vi "MDrive_Get_Parameter.vi"(4 "error in":errorcluster, 6 "Get Parameter":T1, 7 "VISA resource name in":refnum<visa-resource-name>) -> (0 "error out":errorcluster, 1 "Parameter Data Numeric":i32, 2 "Parameter Data String":string, 3 "VISA resource name out":refnum<visa-resource-name>)   [LabVIEW 2013]
uses:
  Get Parameter.ctl
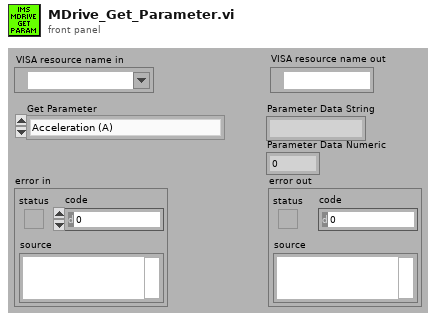
[diagram p1: front panel]
types:
  T1 = typedef "Get Parameter.ctl" = enum16{"Acceleration (A)", "Baud Rate (BD)", "Busy Flag (BY)", "Counter 1 (C1)", "Counter 2 (C2)", "Check Sum Enable (CK)", "Clock Mode (CM)", "Clock Mode Ratio (CR)", "Clock Mode Out Step Width (CW)", "Deceleration (D)", "Digital Filtering, Input 1 (D1)", "Digital Filtering, Input 2 (D2)", "Digital Filtering, Input 3 (D3)", "Digital Filtering, Input 4 (D4)", "Digital Filtering, Input 5 (D5)", "Digital Filtering, Input 9 (D9)", "Digital Filtering, Input 10 (D10)", "Digital Filtering, Input 11 (D11)", "Digital Filtering, Input 12 (D12)", "Deadband (DB)", "Enable/Disable Drive (DE)", "Device Name (DN)", "End Program Execution (E)", "Encoder Function Enable (EE)", "Encoder Lines (EL)", "Error Flag (EF)", "Error Variable (ER)", "Echo Mode (EM)", "Escape (ES)", "Execute Program at Address (EX)", "Hold Current (HC)", "Hold Current Delay Time (HI)", "Input 1 (I1)", "Input 2 (I2)", "Input 3 (I3)", "Input 4 (I4)", "Input 5 Analog (I5)", "Input 6 Encoder Index (I6)", "Input 9 (I9)", "Input 10 (I10)", "Input 11 (I11)", "Input 12 (I12)", "Input Low Byte (1-4) (IL)", "Input High Byte (9-12) (IH)", "Inputs Total (1-4,9-12) (IN)", "Internal Temperature (IT)", "Jog Enable (JE)", "Limit Stop Mode (LM)", "MicroStepping Select (MS)", "Motor Settling Delay Time (MT)", "Moving Flag (MV)", "Output 1 (O1)", "Output 2 (O2)", "Output 3 (O3)", "Output 4 (O4)", "Output 9 (O9)", "Output 10 (O10)", "Output 11 (O11)", "Output 12 (O12)", "Output High Byte (9-12) (OH)", "Output Low Byte (1-4) (OL)", "Output Total (1-4 and 9-12) (OT)", "Position Captured at Trip (PC)", "Position Maintenance (PM)", "Part Number (PN)", "Party Mode (PY)", "Register 1 (R1)", "Register 2 (R2)", "Register 3 (R3)", "Register 4 (R4)", "Run Current (RC)", "Serial Number (SN)", "Stall Flag (ST)", "Stall Factor (SF)", "Stall Mode Set (SM)", "User Variables (UV)", "Velocity (V)", "Velocity Changing Flag (VC)", "Velocity Initial (VI)", "Version, Firmware (VR)", "Velocity Maximum (VM)"}
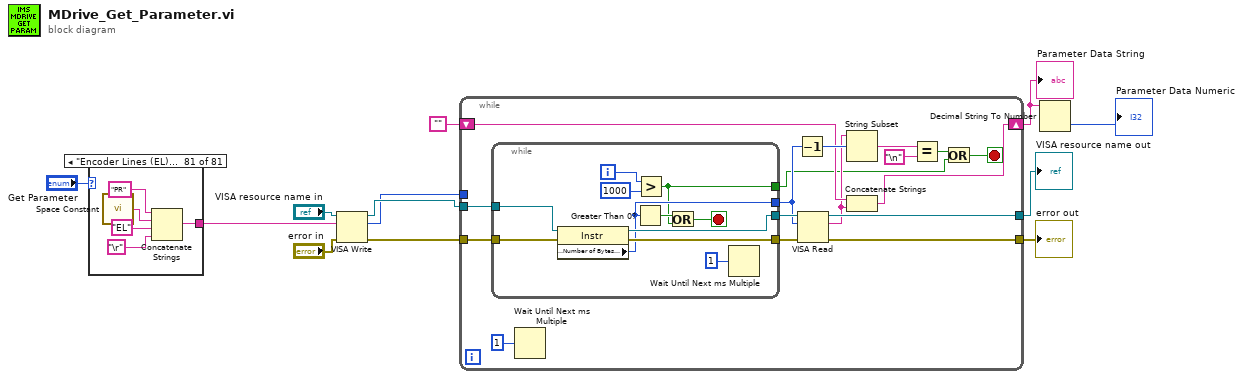
[diagram p0: block diagram]
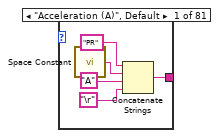
[diagram p2: hidden frame]
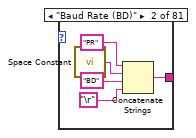
[diagram p3: hidden frame]
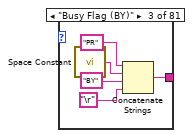
[diagram p4: hidden frame]
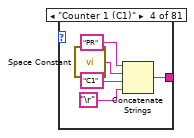
[diagram p5: hidden frame]
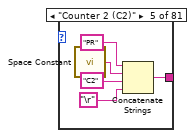
[diagram p6: hidden frame]
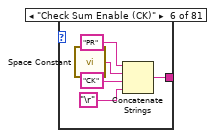
[diagram p7: hidden frame]
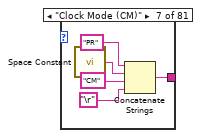
[diagram p8: hidden frame]
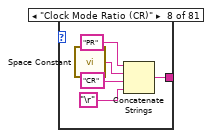
[diagram p9: hidden frame]
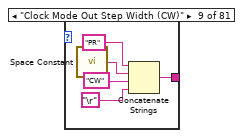
[diagram p10: hidden frame]
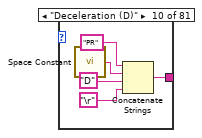
[diagram p11: hidden frame]
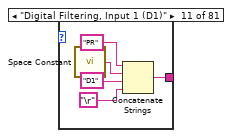
[diagram p12: hidden frame]
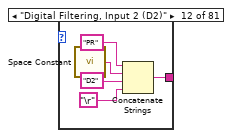
[diagram p13: hidden frame]
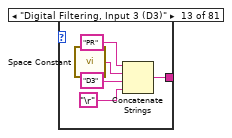
[diagram p14: hidden frame]
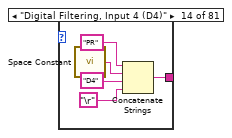
[diagram p15: hidden frame]
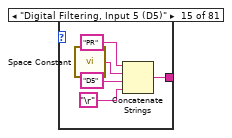
[diagram p16: hidden frame]
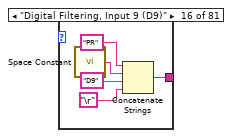
[diagram p17: hidden frame]
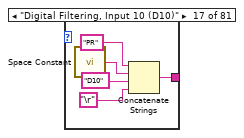
[diagram p18: hidden frame]
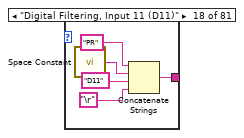
[diagram p19: hidden frame]
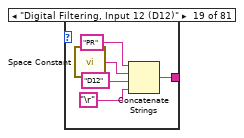
[diagram p20: hidden frame]
diagram:
  n1 = case shown="\"Encoder Lines (EL)\"" "Get Parameter" {
    tunnel: [w13 w18 w23 w28 w33 w38 w43 w48 w53 w58 w63 w68 w73 w78 w83 w88 w93 w98 w103 w108 w113 w118 w123 w128 w133 w138 w143 w148 w153 w158 w163 w168 w173 w178 w183 w188 w193 w198 w203 w208 w213 w218 w223 w228 w233 w238 w243 w248 w253 w258 w263 w268 w273 w278 w283 w288 w293 w298 w303 w308 w313 w318 w323 w328 w333 w338 w343 w348 w353 w358 w363 w368 w373 w378 w383 w388 w393 w398 w403 w408 w413] -> w3
    frame "Acceleration (A)", Default {
      n2 = call <vilib>:"Space Constant.vi"() -> ("String"=w16:string)
      n3 = Concatenate Strings("PR" ("string"), w16, "A" ("string"), "\r") -> (w13:string)
    }
    frame "Baud Rate (BD)" {
      n4 = call <vilib>:"Space Constant.vi"() -> ("String"=w21:string)
      n5 = Concatenate Strings("PR" ("string"), w21, "BD" ("string"), "\r") -> (w18:string)
    }
    frame "Busy Flag (BY)" {
      n6 = call <vilib>:"Space Constant.vi"() -> ("String"=w26:string)
      n7 = Concatenate Strings("PR" ("string"), w26, "BY" ("string"), "\r") -> (w23:string)
    }
    frame "Counter 1 (C1)" {
      n8 = call <vilib>:"Space Constant.vi"() -> ("String"=w31:string)
      n9 = Concatenate Strings("PR" ("string"), w31, "C1" ("string"), "\r") -> (w28:string)
    }
    frame "Counter 2 (C2)" {
      n10 = call <vilib>:"Space Constant.vi"() -> ("String"=w36:string)
      n11 = Concatenate Strings("PR" ("string"), w36, "C2" ("string"), "\r") -> (w33:string)
    }
    frame "Check Sum Enable (CK)" {
      n12 = call <vilib>:"Space Constant.vi"() -> ("String"=w41:string)
      n13 = Concatenate Strings("PR" ("string"), w41, "CK" ("string"), "\r") -> (w38:string)
    }
    frame "Clock Mode (CM)" {
      n14 = call <vilib>:"Space Constant.vi"() -> ("String"=w46:string)
      n15 = Concatenate Strings("PR" ("string"), w46, "CM" ("string"), "\r") -> (w43:string)
    }
    frame "Clock Mode Ratio (CR)" {
      n16 = call <vilib>:"Space Constant.vi"() -> ("String"=w51:string)
      n17 = Concatenate Strings("PR" ("string"), w51, "CR" ("string"), "\r") -> (w48:string)
    }
    frame "Clock Mode Out Step Width (CW)" {
      n18 = call <vilib>:"Space Constant.vi"() -> ("String"=w56:string)
      n19 = Concatenate Strings("PR" ("string"), w56, "CW" ("string"), "\r") -> (w53:string)
    }
    frame "Deceleration (D)" {
      n20 = call <vilib>:"Space Constant.vi"() -> ("String"=w61:string)
      n21 = Concatenate Strings("PR" ("string"), w61, "D" ("string"), "\r") -> (w58:string)
    }
    frame "Digital Filtering, Input 1 (D1)" {
      n22 = call <vilib>:"Space Constant.vi"() -> ("String"=w66:string)
      n23 = Concatenate Strings("PR" ("string"), w66, "D1" ("string"), "\r") -> (w63:string)
    }
    frame "Digital Filtering, Input 2 (D2)" {
      n24 = call <vilib>:"Space Constant.vi"() -> ("String"=w71:string)
      n25 = Concatenate Strings("PR" ("string"), w71, "D2" ("string"), "\r") -> (w68:string)
    }
    frame "Digital Filtering, Input 3 (D3)" {
      n26 = call <vilib>:"Space Constant.vi"() -> ("String"=w76:string)
      n27 = Concatenate Strings("PR" ("string"), w76, "D3" ("string"), "\r") -> (w73:string)
    }
    frame "Digital Filtering, Input 4 (D4)" {
      n28 = call <vilib>:"Space Constant.vi"() -> ("String"=w81:string)
      n29 = Concatenate Strings("PR" ("string"), w81, "D4" ("string"), "\r") -> (w78:string)
    }
    frame "Digital Filtering, Input 5 (D5)" {
      n30 = call <vilib>:"Space Constant.vi"() -> ("String"=w86:string)
      n31 = Concatenate Strings("PR" ("string"), w86, "D5" ("string"), "\r") -> (w83:string)
    }
    frame "Digital Filtering, Input 9 (D9)" {
      n32 = call <vilib>:"Space Constant.vi"() -> ("String"=w91:string)
      n33 = Concatenate Strings("PR" ("string"), w91, "D9" ("string"), "\r") -> (w88:string)
    }
    frame "Digital Filtering, Input 10 (D10)" {
      n34 = call <vilib>:"Space Constant.vi"() -> ("String"=w96:string)
      n35 = Concatenate Strings("PR" ("string"), w96, "D10" ("string"), "\r") -> (w93:string)
    }
    frame "Digital Filtering, Input 11 (D11)" {
      n36 = call <vilib>:"Space Constant.vi"() -> ("String"=w101:string)
      n37 = Concatenate Strings("PR" ("string"), w101, "D11" ("string"), "\r") -> (w98:string)
    }
    frame "Digital Filtering, Input 12 (D12)" {
      n38 = call <vilib>:"Space Constant.vi"() -> ("String"=w106:string)
      n39 = Concatenate Strings("PR" ("string"), w106, "D12" ("string"), "\r") -> (w103:string)
    }
    frame "Deadband (DB)" {
      n40 = call <vilib>:"Space Constant.vi"() -> ("String"=w111:string)
      n41 = Concatenate Strings("PR" ("string"), w111, "DB" ("string"), "\r") -> (w108:string)
    }
    frame "Enable/Disable Drive (DE)" {
      n42 = call <vilib>:"Space Constant.vi"() -> ("String"=w116:string)
      n43 = Concatenate Strings("PR" ("string"), w116, "DE" ("string"), "\r") -> (w113:string)
    }
    frame "Device Name (DN)" {
      n44 = call <vilib>:"Space Constant.vi"() -> ("String"=w121:string)
      n45 = Concatenate Strings("PR" ("string"), w121, "DN" ("string"), "\r") -> (w118:string)
    }
    frame "End Program Execution (E)" {
      n46 = call <vilib>:"Space Constant.vi"() -> ("String"=w126:string)
      n47 = Concatenate Strings("PR" ("string"), w126, "E" ("string"), "\r") -> (w123:string)
    }
    frame "Encoder Function Enable (EE)" {
      n48 = call <vilib>:"Space Constant.vi"() -> ("String"=w131:string)
      n49 = Concatenate Strings("PR" ("string"), w131, "EE" ("string"), "\r") -> (w128:string)
    }
    frame "Error Flag (EF)" {
      n50 = call <vilib>:"Space Constant.vi"() -> ("String"=w136:string)
      n51 = Concatenate Strings("PR" ("string"), w136, "EF" ("string"), "\r") -> (w133:string)
    }
    frame "Error Variable (ER)" {
      n52 = call <vilib>:"Space Constant.vi"() -> ("String"=w141:string)
      n53 = Concatenate Strings("PR" ("string"), w141, "ER" ("string"), "\r") -> (w138:string)
    }
    frame "Echo Mode (EM)" {
      n54 = call <vilib>:"Space Constant.vi"() -> ("String"=w146:string)
      n55 = Concatenate Strings("PR" ("string"), w146, "EM" ("string"), "\r") -> (w143:string)
    }
    frame "Escape (ES)" {
      n56 = call <vilib>:"Space Constant.vi"() -> ("String"=w151:string)
      n57 = Concatenate Strings("PR" ("string"), w151, "ES" ("string"), "\r") -> (w148:string)
    }
    frame "Execute Program at Address (EX)" {
      n58 = call <vilib>:"Space Constant.vi"() -> ("String"=w156:string)
      n59 = Concatenate Strings("PR" ("string"), w156, "EX" ("string"), "\r") -> (w153:string)
    }
    frame "Hold Current (HC)" {
      n60 = call <vilib>:"Space Constant.vi"() -> ("String"=w161:string)
      n61 = Concatenate Strings("PR" ("string"), w161, "HC" ("string"), "\r") -> (w158:string)
    }
    frame "Hold Current Delay Time (HI)" {
      n62 = call <vilib>:"Space Constant.vi"() -> ("String"=w166:string)
      n63 = Concatenate Strings("PR" ("string"), w166, "HI" ("string"), "\r") -> (w163:string)
    }
    frame "Input 1 (I1)" {
      n64 = call <vilib>:"Space Constant.vi"() -> ("String"=w171:string)
      n65 = Concatenate Strings("PR" ("string"), w171, "I1" ("string"), "\r") -> (w168:string)
    }
    frame "Input 2 (I2)" {
      n66 = call <vilib>:"Space Constant.vi"() -> ("String"=w176:string)
      n67 = Concatenate Strings("PR" ("string"), w176, "I2" ("string"), "\r") -> (w173:string)
    }
    frame "Input 3 (I3)" {
      n68 = call <vilib>:"Space Constant.vi"() -> ("String"=w181:string)
      n69 = Concatenate Strings("PR" ("string"), w181, "I3" ("string"), "\r") -> (w178:string)
    }
    frame "Input 4 (I4)" {
      n70 = call <vilib>:"Space Constant.vi"() -> ("String"=w186:string)
      n71 = Concatenate Strings("PR" ("string"), w186, "I4" ("string"), "\r") -> (w183:string)
    }
    frame "Input 5 Analog (I5)" {
      n72 = call <vilib>:"Space Constant.vi"() -> ("String"=w191:string)
      n73 = Concatenate Strings("PR" ("string"), w191, "I5" ("string"), "\r") -> (w188:string)
    }
    frame "Input 6 Encoder Index (I6)" {
      n74 = call <vilib>:"Space Constant.vi"() -> ("String"=w196:string)
      n75 = Concatenate Strings("PR" ("string"), w196, "I6" ("string"), "\r") -> (w193:string)
    }
    frame "Input 9 (I9)" {
      n76 = call <vilib>:"Space Constant.vi"() -> ("String"=w201:string)
      n77 = Concatenate Strings("PR" ("string"), w201, "I9" ("string"), "\r") -> (w198:string)
    }
    frame "Input 10 (I10)" {
      n78 = call <vilib>:"Space Constant.vi"() -> ("String"=w206:string)
      n79 = Concatenate Strings("PR" ("string"), w206, "I10" ("string"), "\r") -> (w203:string)
    }
    frame "Input 11 (I11)" {
      n80 = call <vilib>:"Space Constant.vi"() -> ("String"=w211:string)
      n81 = Concatenate Strings("PR" ("string"), w211, "I3" ("string"), "\r") -> (w208:string)
    }
    frame "Input 12 (I12)" {
      n82 = call <vilib>:"Space Constant.vi"() -> ("String"=w216:string)
      n83 = Concatenate Strings("PR" ("string"), w216, "I12" ("string"), "\r") -> (w213:string)
    }
    frame "Input Low Byte (1-4) (IL)" {
      n84 = call <vilib>:"Space Constant.vi"() -> ("String"=w221:string)
      n85 = Concatenate Strings("PR" ("string"), w221, "IL" ("string"), "\r") -> (w218:string)
    }
    frame "Input High Byte (9-12) (IH)" {
      n86 = call <vilib>:"Space Constant.vi"() -> ("String"=w226:string)
      n87 = Concatenate Strings("PR" ("string"), w226, "IH" ("string"), "\r") -> (w223:string)
    }
    frame "Inputs Total (1-4,9-12) (IN)" {
      n88 = call <vilib>:"Space Constant.vi"() -> ("String"=w231:string)
      n89 = Concatenate Strings("PR" ("string"), w231, "IN" ("string"), "\r") -> (w228:string)
    }
    frame "Internal Temperature (IT)" {
      n90 = call <vilib>:"Space Constant.vi"() -> ("String"=w236:string)
      n91 = Concatenate Strings("PR" ("string"), w236, "IT" ("string"), "\r") -> (w233:string)
    }
    frame "Jog Enable (JE)" {
      n92 = call <vilib>:"Space Constant.vi"() -> ("String"=w241:string)
      n93 = Concatenate Strings("PR" ("string"), w241, "JE" ("string"), "\r") -> (w238:string)
    }
    frame "Limit Stop Mode (LM)" {
      n94 = call <vilib>:"Space Constant.vi"() -> ("String"=w246:string)
      n95 = Concatenate Strings("PR" ("string"), w246, "LM" ("string"), "\r") -> (w243:string)
    }
    frame "MicroStepping Select (MS)" {
      n96 = call <vilib>:"Space Constant.vi"() -> ("String"=w251:string)
      n97 = Concatenate Strings("PR" ("string"), w251, "MS" ("string"), "\r") -> (w248:string)
    }
    frame "Motor Settling Delay Time (MT)" {
      n98 = call <vilib>:"Space Constant.vi"() -> ("String"=w256:string)
      n99 = Concatenate Strings("PR" ("string"), w256, "MT" ("string"), "\r") -> (w253:string)
    }
    frame "Output 1 (O1)" {
      n100 = call <vilib>:"Space Constant.vi"() -> ("String"=w261:string)
      n101 = Concatenate Strings("PR" ("string"), w261, "O1" ("string"), "\r") -> (w258:string)
    }
    frame "Output 2 (O2)" {
      n102 = call <vilib>:"Space Constant.vi"() -> ("String"=w266:string)
      n103 = Concatenate Strings("PR" ("string"), w266, "O2" ("string"), "\r") -> (w263:string)
    }
    frame "Output 3 (O3)" {
      n104 = call <vilib>:"Space Constant.vi"() -> ("String"=w271:string)
      n105 = Concatenate Strings("PR" ("string"), w271, "O3" ("string"), "\r") -> (w268:string)
    }
    frame "Output 4 (O4)" {
      n106 = call <vilib>:"Space Constant.vi"() -> ("String"=w276:string)
      n107 = Concatenate Strings("PR" ("string"), w276, "O4" ("string"), "\r") -> (w273:string)
    }
    frame "Output 9 (O9)" {
      n108 = call <vilib>:"Space Constant.vi"() -> ("String"=w281:string)
      n109 = Concatenate Strings("PR" ("string"), w281, "O9" ("string"), "\r") -> (w278:string)
    }
    frame "Output 10 (O10)" {
      n110 = call <vilib>:"Space Constant.vi"() -> ("String"=w286:string)
      n111 = Concatenate Strings("PR" ("string"), w286, "O10" ("string"), "\r") -> (w283:string)
    }
    frame "Output 11 (O11)" {
      n112 = call <vilib>:"Space Constant.vi"() -> ("String"=w291:string)
      n113 = Concatenate Strings("PR" ("string"), w291, "O11" ("string"), "\r") -> (w288:string)
    }
    frame "Output 12 (O12)" {
      n114 = call <vilib>:"Space Constant.vi"() -> ("String"=w296:string)
      n115 = Concatenate Strings("PR" ("string"), w296, "O12" ("string"), "\r") -> (w293:string)
    }
    frame "Output High Byte (9-12) (OH)" {
      n116 = call <vilib>:"Space Constant.vi"() -> ("String"=w301:string)
      n117 = Concatenate Strings("PR" ("string"), w301, "OH" ("string"), "\r") -> (w298:string)
    }
    frame "Output Low Byte (1-4) (OL)" {
      n118 = call <vilib>:"Space Constant.vi"() -> ("String"=w306:string)
      n119 = Concatenate Strings("PR" ("string"), w306, "OL" ("string"), "\r") -> (w303:string)
    }
    frame "Output Total (1-4 and 9-12) (OT)" {
      n120 = call <vilib>:"Space Constant.vi"() -> ("String"=w311:string)
      n121 = Concatenate Strings("PR" ("string"), w311, "OT" ("string"), "\r") -> (w308:string)
    }
    frame "Position Captured at Trip (PC)" {
      n122 = call <vilib>:"Space Constant.vi"() -> ("String"=w316:string)
      n123 = Concatenate Strings("PR" ("string"), w316, "PC" ("string"), "\r") -> (w313:string)
    }
    frame "Position Maintenance (PM)" {
      n124 = call <vilib>:"Space Constant.vi"() -> ("String"=w321:string)
      n125 = Concatenate Strings("PR" ("string"), w321, "PM" ("string"), "\r") -> (w318:string)
    }
    frame "Part Number (PN)" {
      n126 = call <vilib>:"Space Constant.vi"() -> ("String"=w326:string)
      n127 = Concatenate Strings("PR" ("string"), w326, "PN" ("string"), "\r") -> (w323:string)
    }
    frame "Party Mode (PY)" {
      n128 = call <vilib>:"Space Constant.vi"() -> ("String"=w331:string)
      n129 = Concatenate Strings("PR" ("string"), w331, "PY" ("string"), "\r") -> (w328:string)
    }
    frame "Register 1 (R1)" {
      n130 = call <vilib>:"Space Constant.vi"() -> ("String"=w336:string)
      n131 = Concatenate Strings("PR" ("string"), w336, "R1" ("string"), "\r") -> (w333:string)
    }
    frame "Register 2 (R2)" {
      n132 = call <vilib>:"Space Constant.vi"() -> ("String"=w341:string)
      n133 = Concatenate Strings("PR" ("string"), w341, "R2" ("string"), "\r") -> (w338:string)
    }
    frame "Register 3 (R3)" {
      n134 = call <vilib>:"Space Constant.vi"() -> ("String"=w346:string)
      n135 = Concatenate Strings("PR" ("string"), w346, "R3" ("string"), "\r") -> (w343:string)
    }
    frame "Register 4 (R4)" {
      n136 = call <vilib>:"Space Constant.vi"() -> ("String"=w351:string)
      n137 = Concatenate Strings("PR" ("string"), w351, "R4" ("string"), "\r") -> (w348:string)
    }
    frame "Run Current (RC)" {
      n138 = call <vilib>:"Space Constant.vi"() -> ("String"=w356:string)
      n139 = Concatenate Strings("PR" ("string"), w356, "RC" ("string"), "\r") -> (w353:string)
    }
    frame "Serial Number (SN)" {
      n140 = call <vilib>:"Space Constant.vi"() -> ("String"=w361:string)
      n141 = Concatenate Strings("PR" ("string"), w361, "SN" ("string"), "\r") -> (w358:string)
    }
    frame "Stall Flag (ST)" {
      n142 = call <vilib>:"Space Constant.vi"() -> ("String"=w366:string)
      n143 = Concatenate Strings("PR" ("string"), w366, "ST" ("string"), "\r") -> (w363:string)
    }
    frame "Stall Factor (SF)" {
      n144 = call <vilib>:"Space Constant.vi"() -> ("String"=w371:string)
      n145 = Concatenate Strings("PR" ("string"), w371, "SF" ("string"), "\r") -> (w368:string)
    }
    frame "Stall Mode Set (SM)" {
      n146 = call <vilib>:"Space Constant.vi"() -> ("String"=w376:string)
      n147 = Concatenate Strings("PR" ("string"), w376, "SM" ("string"), "\r") -> (w373:string)
    }
    frame "User Variables (UV)" {
      n148 = call <vilib>:"Space Constant.vi"() -> ("String"=w381:string)
      n149 = Concatenate Strings("PR" ("string"), w381, "UV" ("string"), "\r") -> (w378:string)
    }
    frame "Velocity (V)" {
      n150 = call <vilib>:"Space Constant.vi"() -> ("String"=w386:string)
      n151 = Concatenate Strings("PR" ("string"), w386, "V" ("string"), "\r") -> (w383:string)
    }
    frame "Velocity Changing Flag (VC)" {
      n152 = call <vilib>:"Space Constant.vi"() -> ("String"=w391:string)
      n153 = Concatenate Strings("PR" ("string"), w391, "VC" ("string"), "\r") -> (w388:string)
    }
    frame "Velocity Initial (VI)" {
      n154 = call <vilib>:"Space Constant.vi"() -> ("String"=w396:string)
      n155 = Concatenate Strings("PR" ("string"), w396, "VI" ("string"), "\r") -> (w393:string)
    }
    frame "Version, Firmware (VR)" {
      n156 = call <vilib>:"Space Constant.vi"() -> ("String"=w401:string)
      n157 = Concatenate Strings("PR" ("string"), w401, "VR" ("string"), "\r") -> (w398:string)
    }
    frame "Velocity Maximum (VM)" {
      n158 = call <vilib>:"Space Constant.vi"() -> ("String"=w406:string)
      n159 = Concatenate Strings("PR" ("string"), w406, "VM" ("string"), "\r") -> (w403:string)
    }
    frame "Moving Flag (MV)" {
      n160 = call <vilib>:"Space Constant.vi"() -> ("String"=w411:string)
      n161 = Concatenate Strings("PR" ("string"), w411, "MV" ("string"), "\r") -> (w408:string)
    }
    frame "Encoder Lines (EL)" {
      n162 = call <vilib>:"Space Constant.vi"() -> ("String"=w416:string)
      n163 = Concatenate Strings("PR" ("string"), w416, "EL" ("string"), "\r") -> (w413:string)
    }
  }
  n164 = VISA Write(VISA resource name="VISA resource name in", write buffer=w3, error in (no error)="error in") -> (VISA resource name out=w12:refnum<visa-resource-name>, return count=w8:u32, error out=w11:errorcluster)
  n165 = while {
    tunnel: w12 -> [w432]
    tunnel: w11 -> [w431]
    tunnel: [w430] -> w10
    tunnel: [w429] -> w9
    tunnel: w8 -> [_]
    shift-right: [w422] -> w2
    shift-left: "" -> [w424]
    stop <- w418 stop-if-true
    n166 = while {
      tunnel: [w445] -> w434
      tunnel: [w444] -> w433
      tunnel: w432 -> [w443]
      tunnel: w431 -> [w442]
      tunnel: [w441] -> w427
      tunnel: [w435] -> w419
      i -> [w439]
      stop <- w436 stop-if-true
      n167 = property class="Instr"(reference=w443, error in=w442) -> (reference out=w445:refnum<visa-resource-name>, error out=w444:errorcluster, "Serial Settings:Number of Bytes at Serial Port"=w441:u32)
      n168 = Greater Than 0?(x=w441) -> (x > 0?=w437:bool)
      n169 = Greater?(x=w439, y=1000) -> (0:w435:bool)
      n170 = Or(x=w437, y=w435) -> (x .or. y?=w436:bool)
      n171 = Wait Until Next ms Multiple(millisecond multiple=u32 1) -> ()  [unwired: 1 out]
    }
    n172 = Wait Until Next ms Multiple(millisecond multiple=u32 1) -> ()  [unwired: 1 out]
    n173 = Decrement(x=w427) -> (x-1=w426:u32)
    n174 = VISA Read(VISA resource name=w434, byte count=w427, error in (no error)=w433) -> (VISA resource name out=w430:refnum<visa-resource-name>, read buffer=w423:string, error out=w429:errorcluster)  [unwired: 1 out]
    n175 = String Subset(string=w423, offset (0)=w426) -> (substring=w425:string)  [unwired: 1 in]
    n176 = Concatenate Strings(w424, w423) -> (w422:string)
    n177 = Equal?(x=w425, y="\n") -> (x = y?=w420:bool)
    n178 = Or(x=w420, y=w419) -> (x .or. y?=w418:bool)
  }
  "error out" <- w9
  "VISA resource name out" <- w10
  "Parameter Data String" <- w2
  n179 = Decimal String To Number(string=w2) -> (number=→"Parameter Data Numeric":i32)  [unwired: 2 in, 1 out]
